vi "SetError.vi"(4 "Append timestamp?":bool caption="Append timestamp? (F)", 6 "Error label":string="Custom" caption="Error label (\"Custom\")", 9 "Error in":errorcluster caption="Error in (no error)", 10 "Error description":string caption="Error description (\"\")", 11 "Error code":i32) -> (1 "Error out":errorcluster)   [LabVIEW 2017, in "GPError.lvlib"]
doc: "Sets an error on <B>Error out</B> if <B>Error in</B> allows it.\n\nIf <B>Error in</B> is 'No error' or a warning this VI replaces that with the new error. If <B>Error in</B> is already a collection of appended errors this VI appends the new error to that collection.\n\nThe call chain will always be set in <B>Error out</B> source, and description(s) will be appended from one or more of these sources (in the following order):\n\n1) If any built-in or user defined error/warning descriptions exist in LabVIEW's database these will come first.\n\n2) If any custom descriptions are defined for <B>Error code</B> (with the DefineCustomCode function), these will be appended to the built-in descriptions. If no built-in descriptions exist the custom descriptions are used by themselves.\n\n3) If anything but an empty string is wired to the <B>Error description</B> input this will be appended to any of the above or used by itself if nothing else is defined. This lets you add a final qualifier or give additional info to the specific error on top of the pre-defined, and maybe somewhat generic, descriptions (e.g. \"MyErrorHandler: This error was caused by this specific module not loading due to timeout of X seconds\").\n\nThe optional <B>Error label</B> lets you format the error description for conformity with built-in LabVIEW error messages like this: \"<Label>:\\s\\s<Description>\".\n\nThe optional <B>Append timestamp?</B> specifies if the current UTC time and date will be appended to the source string.\n\nThis VI is inlined.\n\nSteen Schmidt\nGPower\n16/7 2013"
uses:
  GPError.lvlib
  Append/AppendSingle.vi
panel:
  # "Copyright © 2013\nSteen Schmidt, GPower\nSee enclosed license file for terms and conditions"
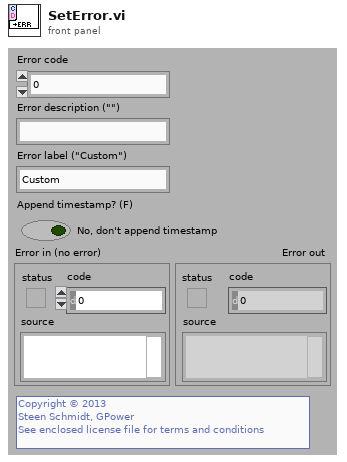
[diagram p1: front panel]
types:
  T1 = typedef "GPError.lvlib/ErrorType.ctl" = enum16{"No Error", "Error", "Warning", "Appended errors", "Appended warnings", "Appended mixed"}
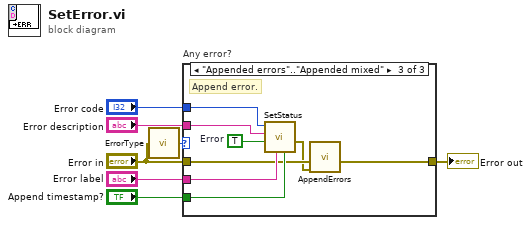
[diagram p0: block diagram]
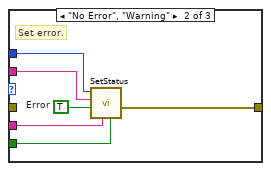
[diagram p3: hidden frame]
diagram:
  n1 = call "ErrorType.vi"("Error in"="Error in") -> ("Error type"=w2:T1)  [unwired: 4 in]
  n2 = case "Any error?" shown="\"Appended errors\"..\"Appended mixed\"" w2 {
    tunnel: [w8 w13 w17] -> w5
    tunnel: "Error code" -> [_ w11 w20]
    tunnel: "Error description" -> [_ w12 w21]
    tunnel: "Append timestamp?" -> [_ w10 w19]
    tunnel: "Error label" -> [_ w9 w18]
    tunnel: "Error in" -> [w8 _ w16]
    frame "Error" {
      # "Keep existing error."
    }
    frame "No Error", "Warning" {
      w14 = TRUE  # Error
      # "Set error."
      n3 = call "SetStatus.vi"("Append timestamp?"=w10, "Label"=w9, "Error?"=w14, "Description"=w12, "Code"=w11) -> ("Error out"=w13:errorcluster)  [unwired: 6 in]
    }
    frame "Appended errors".."Appended mixed" {
      w22 = TRUE  # Error
      # "Append error."
      n4 = call "SetStatus.vi"("Append timestamp?"=w19, "Label"=w18, "Error?"=w22, "Description"=w21, "Code"=w20) -> ("Error out"=w15:errorcluster)  [unwired: 6 in]
      n5 = call-poly "AppendErrors.vi"("Error to append"=w15, "Error in"=w16) -> ("Appended errors out"=w17:errorcluster)  [unwired: 9 in]
    }
  }
  "Error out" <- w5
